vi "Ready_file_Datastorage.vi"(3 "File Path":string, 4 "File save":bool) -> (1 "Ready file created":bool)   [LabVIEW 2024]
uses:
  <vilib>/Utility/file.llb/Write Delimited Spreadsheet (DBL).vi
panel:
  out "error out":errorcluster
  in  "error in (no error)":errorcluster
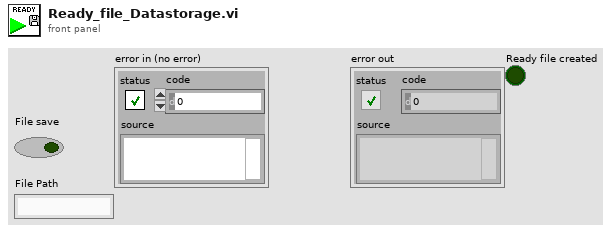
[diagram p1: front panel]
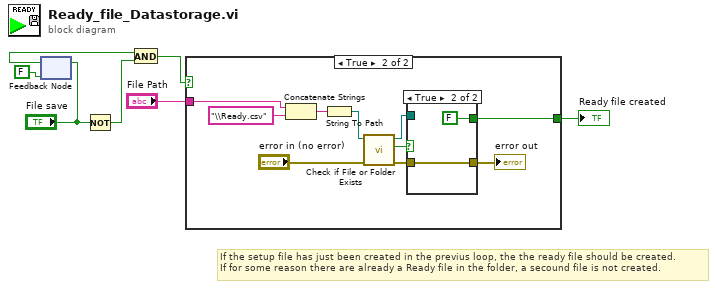
[diagram p0: block diagram]
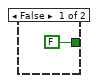
[diagram p2: hidden frame]
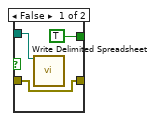
[diagram p3: hidden frame]
diagram:
  # "If the setup file has just been created in the previus loop, the the ready file should be created.\nIf for some reason there are already a Ready file in the folder, a secound file is not created."
  n1 = feedback-in #1("File save") -> ()
  n2 = feedback #1(FALSE) -> (w4:bool)
  n3 = Not(x="File save") -> (.not. x?=w6:bool)
  n4 = And(x=w4, y=w6) -> (x .and. y?=w3:bool)
  n5 = case shown="True" w3 {
    tunnel: "File Path" -> [_ w11]
    tunnel: [FALSE w9] -> w1
    frame False {
    }
    frame True {
      n6 = Concatenate Strings(w11, "\\Ready.csv" ("string")) -> (w12:string)
      n7 = String To Path(string=w12) -> (path=w18:path)
      n8 = call <vilib>:"Check if File or Folder Exists.vi"("error in (no error)"="error in (no error)", "path"=w18) -> ("error out"=w15:errorcluster, "file or folder exists?"=w17:bool, "dup path"=w13:path)  [unwired: 7 in]
      n9 = case shown="True" w17 {
        tunnel: w15 -> [w21 w23]
        tunnel: [w21 w23] -> w14
        tunnel: w13 -> [w20 _]
        tunnel: [TRUE FALSE] -> w9
        frame False {
          n10 = call-poly <vilib>:"Write Delimited Spreadsheet.vi"("file path (dialog if empty)"=w20) -> ()  [unwired: 13 in, 2 out]
        }
        frame True {
        }
      }
      "error out" <- w14
    }
  }
  "Ready file created" <- w1
